vi "Create File List.vi"(8 "error in (no error)":errorcluster, 10 "vi base path":path=path "C:/perforce/Regression/Automation/LabVIEW", 11 "File Path Array in":path[](array[path])) -> (0 "error out":errorcluster, 3 "File Path Array out":path[](array[path]))   [LabVIEW 2012]
panel:
  out "folder names":string[](array[string])
  out "filenames":string[](array[string])
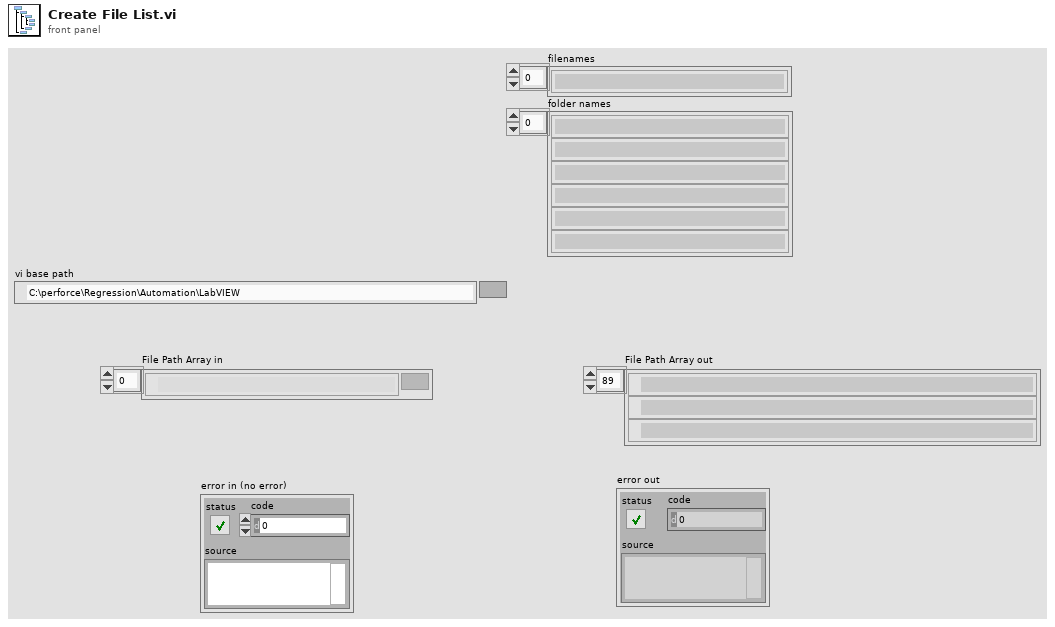
[diagram p1: front panel]
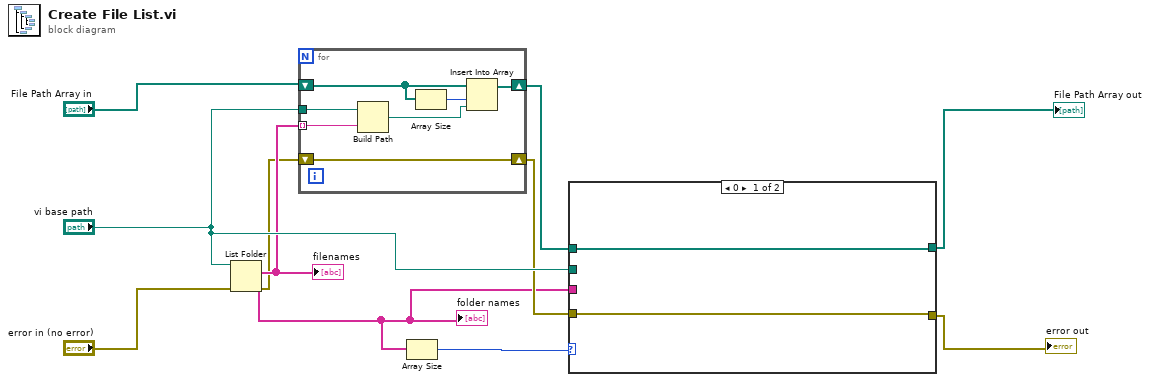
[diagram p0: block diagram]
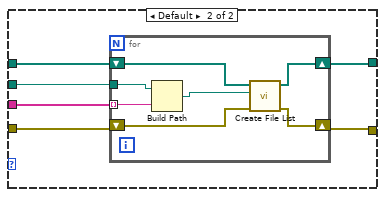
[diagram p2: hidden frame]
diagram:
  n1 = List Folder(path="vi base path", error in="error in (no error)") -> (filenames=w6:string[], folder names=w1:string[], error out=w3:errorcluster)  [unwired: 2 in, 1 out]
  "filenames" <- w6
  "folder names" <- w1
  n2 = for {
    tunnel: "vi base path" -> [w18]
    tunnel: w6 -> [w17] mode=indexing
    shift-right: [w15] -> w4
    shift-left: "File Path Array in" -> [w13]
    shift-right: [w12] -> w2
    shift-left: w3 -> [w12]
    n3 = Build Path(base path=w18, name or relative path=w17) -> (appended path=w16:path)
    n4 = Array Size(array=w13) -> (size(s)=w14:i32)
    n5 = Insert Into Array(array=w13, index=w14, new element=w16) -> (w15:path[])
  }
  n6 = Array Size(array=w1) -> (size(s)=w5:i32)
  n7 = case shown="0" w5 {
    tunnel: w4 -> [w19 w26]
    tunnel: w2 -> [w20 w25]
    tunnel: [w20 w24] -> w7
    tunnel: w1 -> [_ w23]
    tunnel: "vi base path" -> [_ w22]
    tunnel: [w19 w21] -> w9
    frame 0 {
    }
    frame Default {
      n8 = for {
        shift-right: [w30] -> w24
        shift-left: w25 -> [w31]
        shift-right: [w32] -> w21
        shift-left: w26 -> [w33]
        tunnel: w23 -> [w29] mode=indexing
        tunnel: w22 -> [w28]
        n9 = Build Path(base path=w28, name or relative path=w29) -> (appended path=w27:path)
        n10 = call "Create File List.vi"("error in (no error)"=w31, "vi base path"=w27, "File Path Array in"=w33) -> ("error out"=w30:errorcluster, "File Path Array out"=w32:path[])  [unwired: 7 in]
      }
    }
  }
  "File Path Array out" <- w9
  "error out" <- w7
